vi "Generate Sequential String List (DBL).vi"(6 "Precision (3)":i16, 9 "Start Value":dbl, 10 "End Value":dbl, 11 "Number Of Elements":i32) -> (3 "List":string[](array[string]))   [LabVIEW 2015, in "Utility.lvlib"]
uses:
  Utility.lvlib
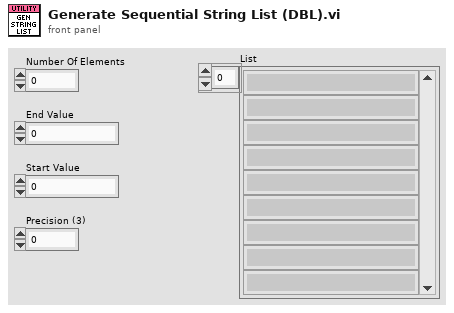
[diagram p1: front panel]
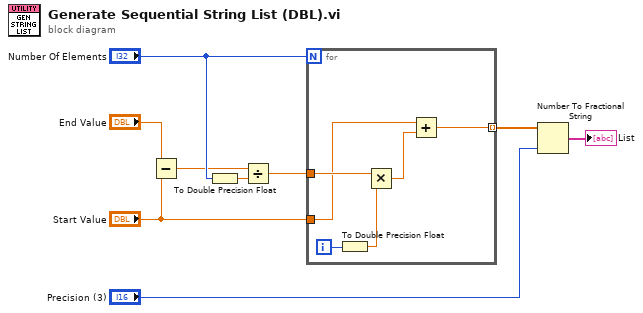
[diagram p0: block diagram]
diagram:
  n1 = Subtract(x="End Value", y="Start Value") -> (x-y=w5:dbl)
  n2 = To Double Precision Float(number="Number Of Elements") -> (double precision float=w7:dbl)
  n3 = Divide(x=w5, y=w7) -> (x/y=w8:dbl)
  n4 = for {
    N: "Number Of Elements" -> [_]
    tunnel: "Start Value" -> [w10]
    tunnel: w8 -> [w11]
    tunnel: [w12] -> w9 mode=indexing
    i -> [w15]
    n5 = To Double Precision Float(number=w15) -> (double precision float=w14:dbl)
    n6 = Multiply(x=w11, y=w14) -> (x*y=w13:dbl)
    n7 = Add(x=w10, y=w13) -> (x+y=w12:dbl)
  }
  n8 = Number To Fractional String(number=w9, precision (6)="Precision (3)") -> (F-format string=→"List":string[])  [unwired: 2 in]
